vi "update last messages.vi"(8 "error in (no error)":errorcluster, 11 "Header content in":refnum<class "Header content.lvclass">) -> (0 "error out":errorcluster, 3 "Header content out":refnum<class "Header content.lvclass">)   [LabVIEW 2018, in "Header content.lvclass"]
uses:
  Header content.lvclass
  Header content.lvclass/Header content.ctl
  Server/Server.lvclass
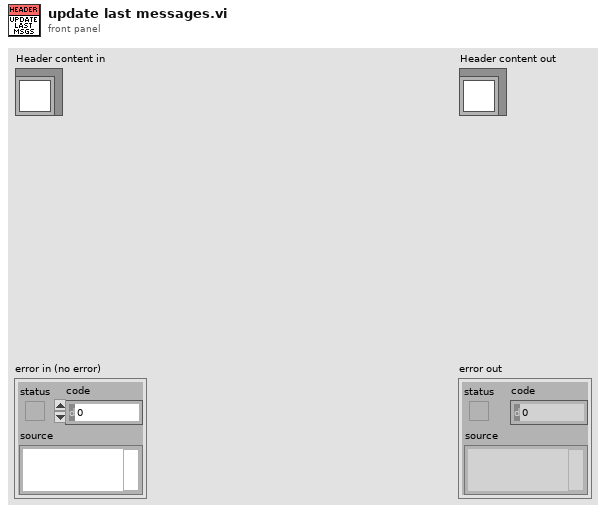
[diagram p1: front panel]
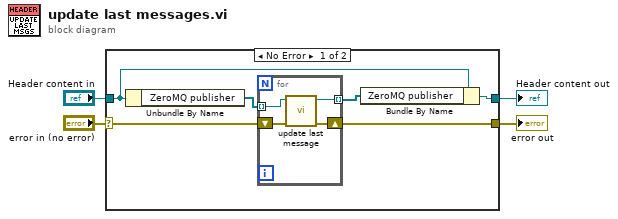
[diagram p0: block diagram]
diagram:
  n1 = case shown="No Error" "error in (no error)" {
    selector: "error in (no error)" -> [w9 w16]
    tunnel: [w8 w16] -> w3
    tunnel: [w6 w15] -> w1
    tunnel: "Header content in" -> [w7 w15]
    frame No Error {
      n2 = Unbundle By Name(w7) -> ("ZeroMQ publisher"=w10:refnum<class "Server.lvclass">[])
      n3 = for {
        tunnel: w10 -> [w11] mode=indexing
        shift-right: [w14] -> w8
        shift-left: w9 -> [w12]
        tunnel: [w13] -> w5 mode=indexing
        n4 = call "update last message.vi"("error in (no error)"=w12, "Server in"=w11) -> ("error out"=w14:errorcluster, "Server out"=w13:refnum<class "Server.lvclass">)  [unwired: 8 in]
      }
      n5 = Bundle By Name(cluster=w7, "ZeroMQ publisher"=w5) -> (w6:refnum<class "Header content.lvclass">)
    }
    frame Error {
    }
  }
  "error out" <- w3
  "Header content out" <- w1
